vi "InsertNode.vi"(8 "error in (no error)":errorcluster, 11 "LLSearch in":refnum<class "LLSearch.lvclass">) -> (0 "error out":errorcluster, 3 "LLSearch out":refnum<class "LLSearch.lvclass">)   [LabVIEW 2009, in "LLSearch.lvclass"]
uses:
  LLSearch.lvclass
  LLNode/LLNode.lvclass
panel:
  out "LLNode out":refnum<data-value>
  in  "LLNode in":refnum<data-value>
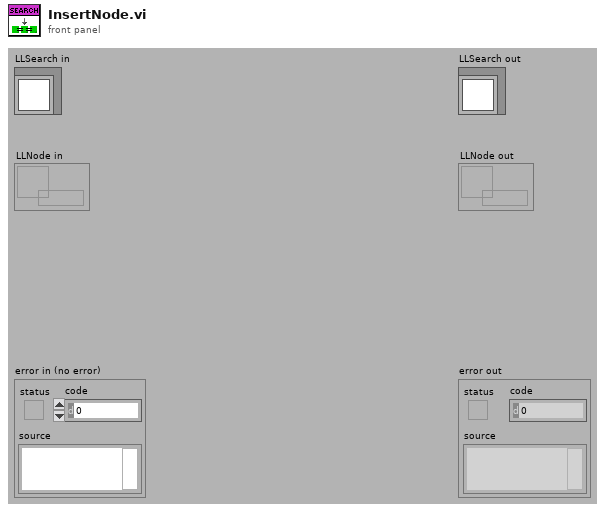
[diagram p1: front panel]
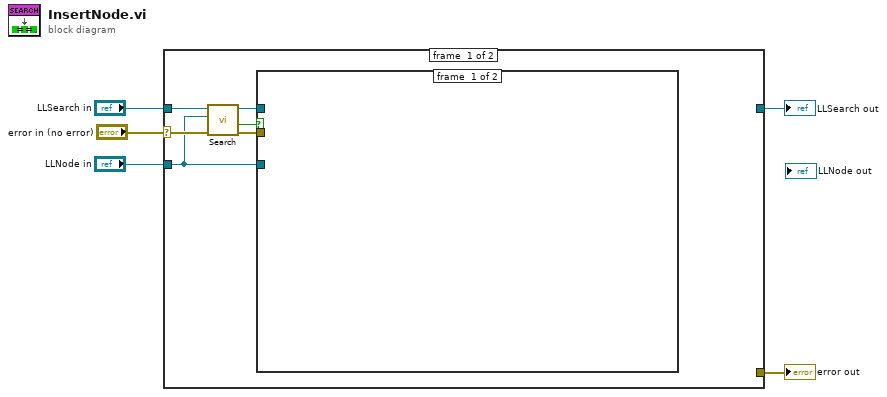
[diagram p0: block diagram]
diagram:
  n1 = case shown="No Error" "error in (no error)" {
    selector: "error in (no error)" -> [w10 w13]
    tunnel: [_ w13] -> w4
    tunnel: [_ w12] -> w2
    tunnel: "LLSearch in" -> [w11 w12]
    tunnel: "LLNode in" -> [w6 _]
    frame #0 {
      n2 = call "Search.vi"("error in (no error)"=w10, "LLNode in"=w6, "LLSearch in"=w11) -> ("error out"=w8:errorcluster, "found"=w9:bool, "LLSearch out"=w7:refnum<class "LLSearch.lvclass">)  [unwired: 5 in, 1 out]
      n3 = case shown="True" w9 {
        tunnel: w8 -> [_ _]
        tunnel: w7 -> [_ _]
        tunnel: w6 -> [_ _]
        frame #0 {
        }
        frame #1 {
        }
      }
    }
    frame #1 {
    }
  }
  "error out" <- w4
  "LLSearch out" <- w2
